vi "I3C Generator.vi"(5 "duration":dbl, 6 "I3C amplitude":dbl, 7 "I3C Generator Fgen Channel":string, 8 "error in (no error)":errorcluster, 9 "I3C frequency":dbl, 10 "I3C waveform":T1(ring), 11 "IVI Refnum in":refnum<k15>) -> (0 "error out":errorcluster, 3 "Numeric":dbl)   [LabVIEW 2021, in "Waveform Generator T1.lvlib"]
uses:
  Waveform Generator T1.lvlib
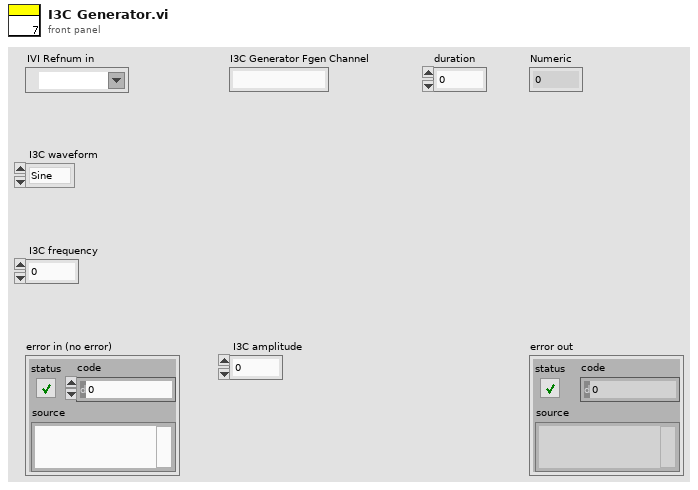
[diagram p1: front panel]
types:
  T1 = enum32{"Sine", "Square", "Triangle", "Ramp Up", "Ramp Down", "DC", "Noise", "User"}
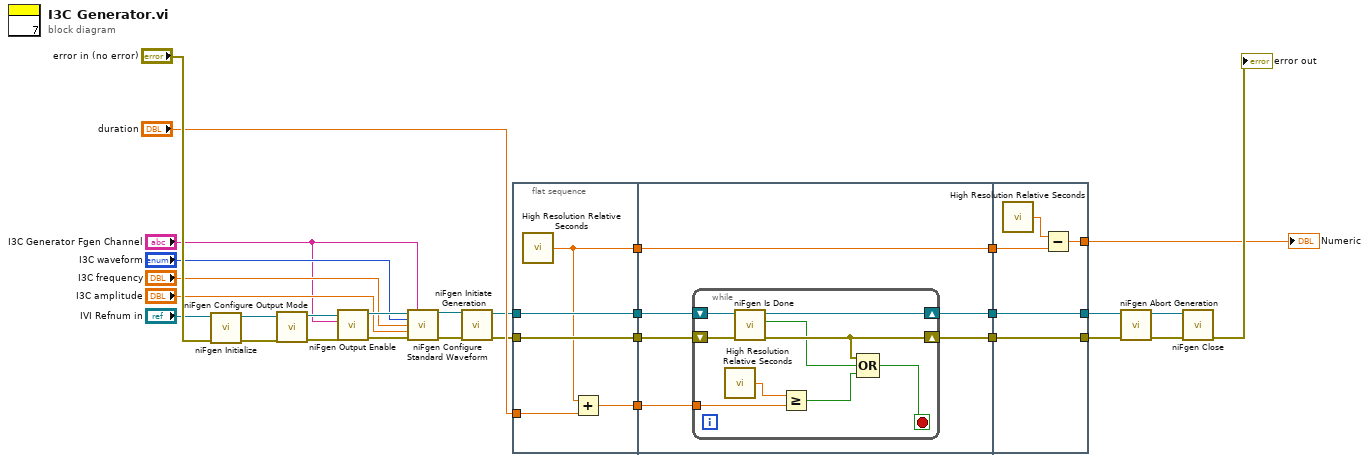
[diagram p0: block diagram]
diagram:
  n1 = call <instrlib>:"niFgen Initialize.vi"("error in (no error)"="error in (no error)", "Resource Name"="IVI Refnum in") -> ("error out"=w17:errorcluster, "Instrument Handle Out"=w20:refnum<k15>)  [unwired: 8 in]
  n2 = call <instrlib>:"niFgen Configure Output Mode.vi"("error in (no error)"=w17, "Instrument Handle"=w20) -> ("error out"=w7:errorcluster, "Instrument Handle Out"=w16:refnum<k15>)  [unwired: 7 in]
  n3 = call <instrlib>:"niFgen Output Enable.vi"("error in (no error)"=w7, "Channel Name"="I3C Generator Fgen Channel", "Instrument Handle"=w16) -> ("error out"=w18:errorcluster, "Instrument Handle Out"=w15:refnum<k15>)  [unwired: 7 in]
  n4 = call <instrlib>:"niFgen Configure Standard Waveform.vi"("Instrument Handle"=w15, "Channel Name"="I3C Generator Fgen Channel", "Waveform"="I3C waveform", "Frequency"="I3C frequency", "Amplitude"="I3C amplitude", "error in (no error)"=w18) -> ("Instrument Handle Out"=w14:refnum<k15>, "error out"=w19:errorcluster)  [unwired: 8 in]
  n5 = call <instrlib>:"niFgen Initiate Generation.vi"("error in (no error)"=w19, "Instrument Handle"=w14) -> ("error out"=w11:errorcluster, "Instrument Handle Out"=w13:refnum<k15>)  [unwired: 8 in]
  n6 = flat-sequence {
    tunnel: w11 -> [w34]
    tunnel: w13 -> [w35]
    tunnel: [w35] -> w30
    tunnel: [w34] -> w29
    tunnel: [w33] -> w28
    tunnel: "duration" -> [w32]
    tunnel: [w31] -> w27
    tunnel: w30 -> [w41]
    tunnel: w29 -> [w39]
    tunnel: [w40] -> w26
    tunnel: [w38] -> w25
    tunnel: [w37] -> w24
    tunnel: w28 -> [w37]
    tunnel: w27 -> [w36]
    tunnel: [w54] -> w10
    tunnel: [w55] -> w12
    tunnel: w26 -> [w55]
    tunnel: w25 -> [w54]
    tunnel: w24 -> [w52]
    tunnel: [w51] -> w1
    frame #0 {
      n7 = call <vilib>:"High Resolution Relative Seconds.vi"() -> ("relative seconds"=w33:dbl)
      n8 = Add(x=w33, y=w32) -> (x+y=w31:dbl)
    }
    frame #1 {
      n9 = while {
        shift-right: [w49] -> w40
        shift-left: w41 -> [w50]
        shift-right: [w47] -> w38
        shift-left: w39 -> [w48]
        tunnel: w36 -> [w44]
        stop <- w46 stop-if-true
        n10 = call <vilib>:"High Resolution Relative Seconds.vi"() -> ("relative seconds"=w45:dbl)
        n11 = call <instrlib>:"niFgen Is Done.vi"("error in (no error)"=w48, "Instrument Handle"=w50) -> ("error out"=w47:errorcluster, "Done"=w42:bool, "Instrument Handle Out"=w49:refnum<k15>)  [unwired: 7 in]
        n12 = Greater Or Equal?(x=w45, y=w44) -> (x >= y?=w43:bool)
        n13 = Compound Arithmetic op=OR(w47, w42, w43) -> (w46:bool)
      }
    }
    frame #2 {
      n14 = call <vilib>:"High Resolution Relative Seconds.vi"() -> ("relative seconds"=w53:dbl)
      n15 = Subtract(x=w53, y=w52) -> (x-y=w51:dbl)
    }
  }
  n16 = call <instrlib>:"niFgen Abort Generation.vi"("error in (no error)"=w10, "Instrument Handle"=w12) -> ("error out"=w8:errorcluster, "Instrument Handle Out"=w9:refnum<k15>)  [unwired: 8 in]
  n17 = call <instrlib>:"niFgen Close.vi"("error in (no error)"=w8, "Instrument Handle"=w9) -> ("error out"=→"error out":errorcluster)  [unwired: 9 in]
  "Numeric" <- w1
